vi "WB_255_int_random_gen_sub_양수만.vi"() -> (1 "number":i64, 2 "배열":i64[][](array[numeric]))   [LabVIEW 2021]
uses:
  <vilib>/numeric/Random Number (Range) I64.vi
  <vilib>/numeric/sub_Random U32.vi
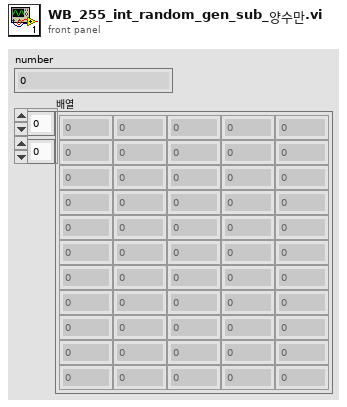
[diagram p1: front panel]
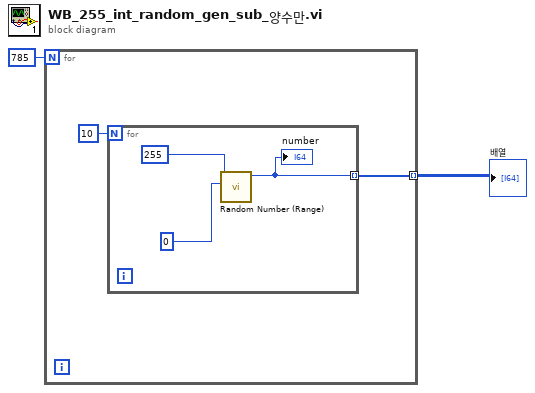
[diagram p0: block diagram]
diagram:
  n1 = for {
    N: 785 -> [_]
    tunnel: [w3] -> w1 mode=indexing
    n2 = for {
      N: 10 -> [_]
      tunnel: [w5] -> w3 mode=indexing
      n3 = call-poly <vilib>:"Random Number (Range).vi"("lower bound (-100)"=i64 0, "upper bound (100)"=i64 255) -> ("number"=w5:i64)  [unwired: 9 in]
      "number" <- w5
    }
  }
  "배열" <- w1
